vi "Read Font from PDF Report.vi"(0 "PDF Report":refnum<class "PDF Report Class.lvclass">, 11 "error in (no error)":errorcluster) -> (2 "Font Class.lvclass":refnum<class "Font Class.lvclass">, 4 "PDF Report duplicate":refnum<class "PDF Report Class.lvclass">, 6 "Font OUT":T2={"Name"="Helvetica", "Size"=12.0, "Color"=0, "Style"={"Bold"=FALSE, "Italic"=FALSE, "Underline"=FALSE, "Strikeout"=FALSE}, "Type"={"Type&direction"=enum."Select", "Embedded"=FALSE, "Encoding"=""}}, 8 "System Fonts":T1, 10 "Font Ref":refnum<k24>, 14 "Font Size":T3=18.0, 15 "error out":errorcluster)   [LabVIEW 2019, in "Font Class.lvclass"]
doc: "Version 1.0\nDeveloped by Jean-Marc Simard\nCopyright © 2010, Exaprom Inc.\nAll rights reserved.\nLicense: BSD\n\nWith iTextSharp 4.1.6 (http://itextsharp.sourceforge.net)\nunder Mozilla Public License Version 1.1\n(http://www.mozilla.org/MPL/MPL-1.1.html)"
uses:
  <userlib>/Exaprom PDF/LV Class/Fonts Class/Font Class.lvclass
  <userlib>/Exaprom PDF/LV Class/PDF Report Class/PDF Report Class.lvclass
  C:/Program Files/National Instruments/LabVIEW 2019/user.lib/Exaprom PDF/DLL/itextsharp.dll
  DLL/itextsharp.dll
  <userlib>/Exaprom PDF/Controls/Font Controls/Font size.ctl
  <userlib>/Exaprom PDF/Controls/Font Controls/Font complete cluster.ctl
  <userlib>/Exaprom PDF/Controls/Font Controls/Font color.ctl
  <userlib>/Exaprom PDF/Controls/Font Controls/Type and encoding.ctl
  <userlib>/Exaprom PDF/Controls/Text Controls/Unicode/Type and run direction.ctl
  <userlib>/Exaprom PDF/Controls/Font Controls/System Fonts.ctl
  <userlib>/Exaprom PDF/LV Class/Fonts Class/Font Class.lvclass/Font Class.ctl
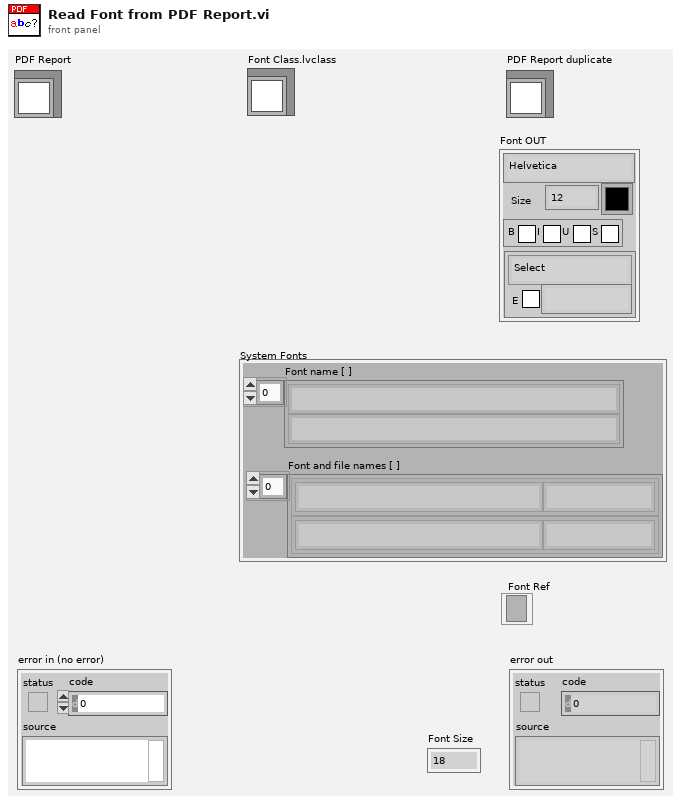
[diagram p1: front panel]
types:
  T1 = typedef "System Fonts.ctl" = cluster{"Font name [ ]":string[], "Font and file names [ ]":cluster{"Font name":string, "File name":string}[]}
  T2 = typedef "Font complete cluster.ctl" = cluster{"Name":string, "Size":T3, "Color":T4, "Style":cluster{"Bold":bool, "Italic":bool, "Underline":bool, "Strikeout":bool}, "Type":T5}
  T3 = typedef "Font size.ctl" = sgl
  T4 = typedef "Font color.ctl" = u32
  T5 = typedef "Type and encoding.ctl" = cluster{"Type&direction":T6, "Embedded":bool, "Encoding":string}
  T6 = typedef "Type and run direction.ctl" = enum16{"Select", "ASCII", "UTF-16", "UTF-16 (default)", "UTF-16 (LTR)", "UTF-16 (RTL)"}
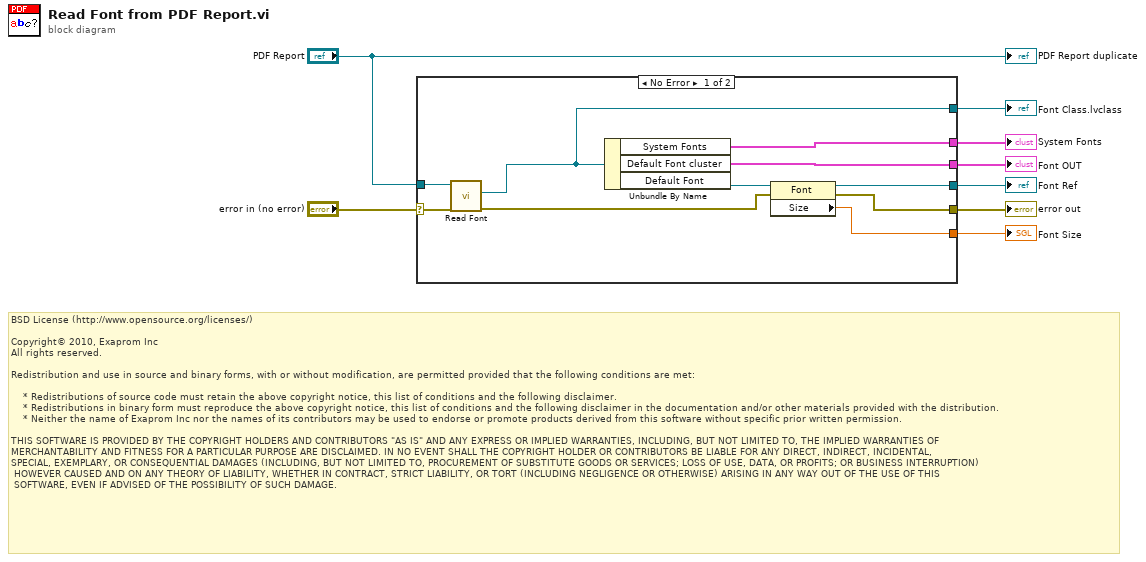
[diagram p0: block diagram]
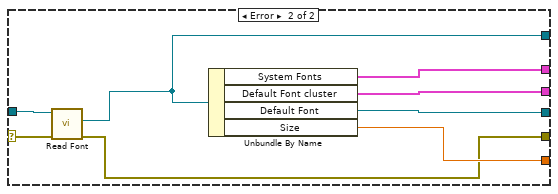
[diagram p2: hidden frame]
diagram:
  # "BSD License (http://www.opensource.org/licenses/)\n\nCopyright© 2010, Exaprom Inc\nAll rights reserved.\n\nRedistribution and use in source and binary forms, with or without modification, are permitted provided that the following conditions are met:\n\n    * Redistributions of source code must retain the above copyright notice, this list of conditions and the following disclaimer.\n    * Redistributions in binary form must reproduce the above copyright notice, this list of conditions and the following disclaimer in the documentation and/or other materials provided with the distribution.\n    * Neither the name of Exaprom Inc nor the names of its contributors may be used to endorse or promote products derived from this software without specific prior written permission.\n\nTHIS SOFTWARE IS PROVIDED BY THE COPYRIGHT HOLDERS AND CONTRIBUTORS \"AS IS\" AND ANY EXPRESS OR IMPLIED WARRANTIES, INCLUDING, BUT NOT LIMITED TO, THE IMPLIED WARRANTIES OF \nMERCHANTABILITY AND FITNESS FOR A PARTICULAR PURPOSE ARE DISCLAIMED. IN NO EVENT SHALL THE COPYRIGHT HOLDER OR CONTRIBUTORS BE LIABLE FOR ANY DIRECT, INDIRECT, INCIDENTAL,\nSPECIAL, EXEMPLARY, OR CONSEQUENTIAL DAMAGES (INCLUDING, BUT NOT LIMITED TO, PROCUREMENT OF SUBSTITUTE GOODS OR SERVICES; LOSS OF USE, DATA, OR PROFITS; OR BUSINESS INTERRUPTION)\n HOWEVER CAUSED AND ON ANY THEORY OF LIABILITY, WHETHER IN CONTRACT, STRICT LIABILITY, OR TORT (INCLUDING NEGLIGENCE OR OTHERWISE) ARISING IN ANY WAY OUT OF THE USE OF THIS\n SOFTWARE, EVEN IF ADVISED OF THE POSSIBILITY OF SUCH DAMAGE."
  n1 = case shown="No Error" "error in (no error)" {
    selector: "error in (no error)" -> [w9 w20]
    tunnel: [w18 w19] -> w8
    tunnel: [w17 w23] -> w7
    tunnel: [w14 w26] -> w6
    tunnel: "PDF Report" -> [w12 w21]
    tunnel: [w16 w24] -> w4
    tunnel: [w13 w25] -> w2
    tunnel: [w11 w22] -> w1
    frame No Error {
      n2 = call-dynamic "Read Font.vi"("error in (no error)"=w9, "PDF Report Class in"=w12) -> ("error out"=w10:errorcluster, "Font Class.lvclass"=w11:refnum<class "Font Class.lvclass">)  [unwired: 7 in, 1 out]
      n3 = Unbundle By Name(w11) -> ("System Fonts"=w13:T1, "Default Font cluster"=w14:T2, "Default Font"=w15:refnum<k24>)
      n4 = property class="Font"(reference=w15, error in=w10) -> (reference out=w17:refnum<k24>, error out=w18:errorcluster, "Size"=w16:sgl)
    }
    frame Error {
      n5 = call-dynamic "Read Font.vi"("error in (no error)"=w20, "PDF Report Class in"=w21) -> ("error out"=w19:errorcluster, "Font Class.lvclass"=w22:refnum<class "Font Class.lvclass">)  [unwired: 7 in, 1 out]
      n6 = Unbundle By Name(w22) -> ("System Fonts"=w25:T1, "Default Font cluster"=w26:T2, "Default Font"=w23:refnum<k24>, "Size"=w24:T3)
    }
  }
  "error out" <- w8
  "Font Ref" <- w7
  "Font Size" <- w4
  "Font OUT" <- w6
  "System Fonts" <- w2
  "Font Class.lvclass" <- w1
  "PDF Report duplicate" <- "PDF Report"
